vi "LinearFilter_SinglePoleIIR.vi"(9 "SamplePeriod":dbl format="%13.5p", 11 "TimeConstant":dbl format="%13.5p") -> (1 "Cutoff Freq":dbl format="%13.5p", 3 "LINEAR_FILTER":T1 {"Outputs" format="%13.5g"; "Inputs" format="%13.5g"; "OutputGains" format="%13.5g"; "InputGains" format="%13.5g"})   [LabVIEW 2019, in "Trajectory_Library.lvlib"]
doc: "Creates a one-pole IIR low-pass filter of the form: \n\n y[n] = (1-gain)*x[n] + gain*y[n-1] \n\n where \n gain = e^(-dt / T), \n T is the time constant in seconds.\n \nThis filter is stable for time constants greater than zero.\n\nInputs: \n - timeConstant - The discrete-time time constant in seconds.\n -samplePeriod - The period in seconds between samples taken by the user.\n\nOutputs:\n - Linearfilter - Created datat structure\n - Cutoff Frequency - Frequency (Hz)"
uses:
  Trajectory_Library.lvlib
  TypeDef/LINEAR_FILTER.ctl
  <vilib>/Rock Robotics/SystemInterfaces/NetworkCommunication/NetComm_UsageReport_report.vi
  Globals/Util_LibraryGlobals.vi
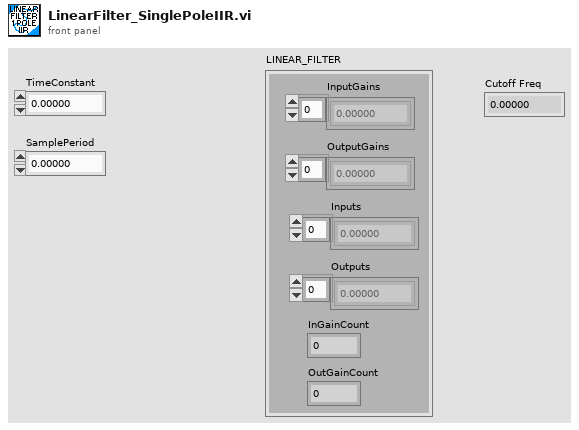
[diagram p1: front panel]
types:
  T1 = typedef "Trajectory_Library.lvlib/LINEAR_FILTER.ctl" = cluster{"InputGains":dbl[], "OutputGains":dbl[], "Inputs":dbl[], "Outputs":dbl[], "InGainCount":i32, "OutGainCount":i32}
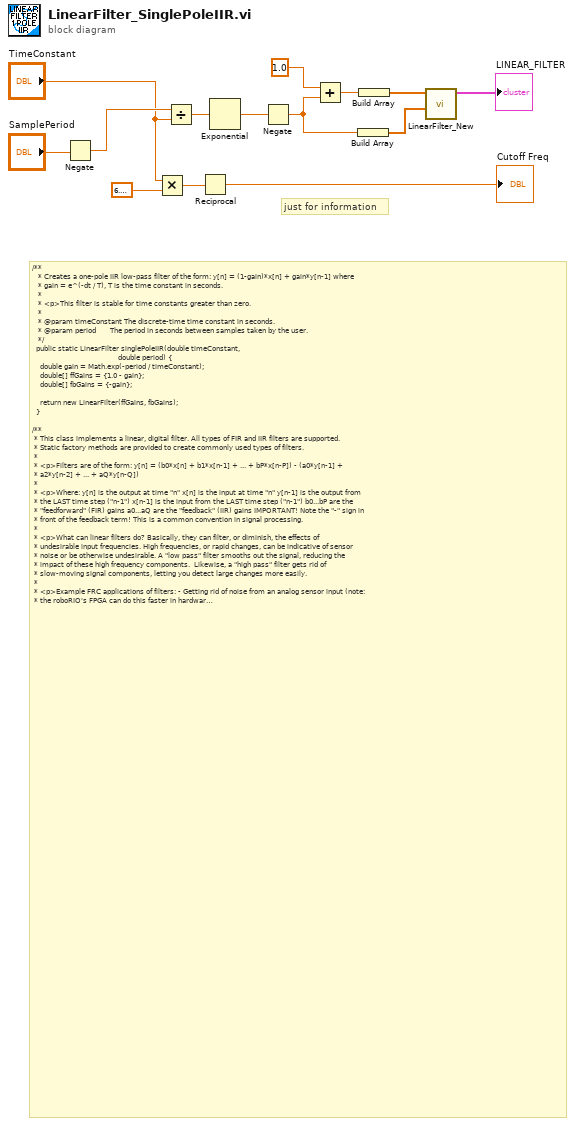
[diagram p0: block diagram]
diagram:
  # "just for information"
  # "/**\n   * Creates a one-pole IIR low-pass filter of the form: y[n] = (1-gain)*x[n] + gain*y[n-1] where\n   * gain = e^(-dt / T), T is the time constant in seconds.\n   *\n   * <p>This filter is stable for time constants greater than zero.\n   *\n   * @param timeConstant The discrete-time time constant in seconds.\n   * @param period       The period in seconds between samples taken by the user.\n   */\n  public static LinearFilter singlePoleIIR(double timeConstant,\n                                           double period) {\n    double gain = Math.exp(-period / timeConstant);\n    double[] ffGains = {1.0 - gain};\n    double[] fbGains = {-gain};\n\n    return new LinearFilter(ffGains, fbGains);\n  }\n\n/**\n * This class implements a linear, digital filter. All types of FIR and IIR filters are supported.\n * Static factory methods are provided to create commonly used types of filters.\n *\n * <p>Filters are of the form: y[n] = (b0*x[n] + b1*x[n-1] + ... + bP*x[n-P]) - (a0*y[n-1] +\n * a2*y[n-2] + ... + aQ*y[n-Q])\n *\n * <p>Where: y[n] is the output at time \"n\" x[n] is the input at time \"n\" y[n-1] is the output from\n * the LAST time step (\"n-1\") x[n-1] is the input from the LAST time step (\"n-1\") b0...bP are the\n * \"feedforward\" (FIR) gains a0...aQ are the \"feedback\" (IIR) gains IMPORTANT! Note the \"-\" sign in\n * front of the feedback term! This is a common convention in signal processing.\n *\n * <p>What can linear filters do? Basically, they can filter, or diminish, the effects of\n * undesirable input frequencies. High frequencies, or rapid changes, can be indicative of sensor\n * noise or be otherwise undesirable. A \"low pass\" filter smooths out the signal, reducing the\n * impact of these high frequency components.  Likewise, a \"high pass\" filter gets rid of\n * slow-moving signal components, letting you detect large changes more easily.\n *\n * <p>Example FRC applications of filters: - Getting rid of noise from an analog sensor input (note:\n * the roboRIO's FPGA can do this faster in hardware) - Smoothing out joystick input to prevent the\n * wheels from slipping or the robot from tipping - Smoothing motor commands so that unnecessary\n * strain isn't put on electrical or mechanical components - If you use clever gains, you can make a\n * PID controller out of this class!\n *\n * <p>For more on filters, we highly recommend the following articles:<br>\n * https://en.wikipedia.org/wiki/Linear_filter<br>\n * https://en.wikipedia.org/wiki/Iir_filter<br>\n * https://en.wikipedia.org/wiki/Fir_filter<br>\n *\n * <p>Note 1: calculate() should be called by the user on a known, regular period. You can use a\n * Notifier for this or do it \"inline\" with code in a periodic function.\n *\n * <p>Note 2: For ALL filters, gains are necessarily a function of frequency. If you make a filter\n * that works well for you at, say, 100Hz, you will most definitely need to adjust the gains if you\n * then want to run it at 200Hz! Combining this with Note 1 - the impetus is on YOU as a developer\n * to make sure calculate() gets called at the desired, constant frequency!\n */"
  n1 = Negate(x="SamplePeriod") -> (-x=w5:dbl)
  n2 = Multiply(x="TimeConstant", y=6.283185307179586) -> (x*y=w2:dbl)
  n3 = Divide(x=w5, y="TimeConstant") -> (x/y=w13:dbl)
  n4 = Reciprocal(x=w2) -> (1/x=→"Cutoff Freq":dbl)
  n5 = Exponential(1:w13) -> (0:w11:dbl)
  n6 = Negate(x=w11) -> (-x=w9:dbl)
  n7 = Add(x=1.0, y=w9) -> (x+y=w10:dbl)
  n8 = Build Array(w9) -> (w7:dbl[])
  n9 = Build Array(w10) -> (w8:dbl[])
  n10 = call "LinearFilter_New.vi"("OutputGains"=w7, "InputGains"=w8) -> ("LINEAR_FILTER"=→"LINEAR_FILTER":T1)  [unwired: 9 in]
